vi "Obtain ACQ Data Notifier.vi"(8 "error in (no error)":errorcluster) -> (0 "error out":errorcluster, 3 "ACQ Data Notifier out":refnum<notifier>)   [LabVIEW 2014, in "WINFAS 2 Data Queue.lvlib"]
uses:
  WINFAS 2 Data Queue.lvlib
  Acquisition Data 1 Sample Cluster.ctl
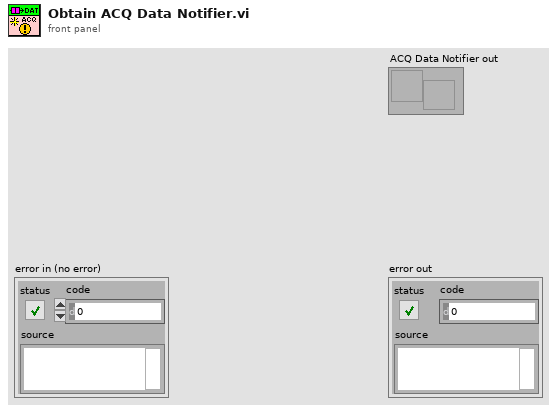
[diagram p1: front panel]
types:
  T1 = typedef "WINFAS 2 Data Queue.lvlib/Acquisition Data 1 Sample Cluster.ctl" = cluster{"TDX":sgl[], "Encoder":sgl}
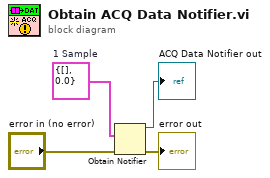
[diagram p0: block diagram]
diagram:
  w2 = T1 {"TDX"=[], "Encoder"=0.0}  # 1 Sample
  n1 = Obtain Notifier(notification data type=w2, error in (no error)="error in (no error)") -> (notifier out=→"ACQ Data Notifier out":refnum<notifier>, error out=→"error out":errorcluster)  [unwired: 2 in, 1 out]
